vi "4Pi Focus Lock_ids.vi"() -> ()   [LabVIEW 2016]
uses:
  4Pi Focus Lock Controls/4Pi Focus Lock - Notifier Type.ctl
  4Pi Focus Lock Controls/4Pi Focus Lock - Actions.ctl
  <vilib>/vision/Image Controls.llb/IMAQ Image.ctl
  Hardware Configuration/Hardware Configuration Controls/Device Type.ctl
  Hardware Configuration/Hardware Configuration Controls/Device Function.ctl
  Device Library/Cameras/Camera Controls/Generic Camera ROI.ctl
  Device Library/Cameras/Camera Controls/Generic Camera Actions.ctl
  Device Library/Stages/Stages Controls/Stage Actions.ctl
  <vilib>/addons/control/pid/pid.llb/PID (DBL).vi
  <vilib>/addons/control/pid/NI_PID_pid.lvlib
  <vilib>/vision/NI_Vision_Development_Module.lvlib
panel:
  out "CC Max":cluster{" cc max":dbl}(graph)
  in  "Pixe Size (µm)":dbl=1.0
  out "X Y Fit Value (µm)":cluster{dbl, dbl, dbl}(graph)
  out "cc max":dbl=1.0 format="%.3g"
  out "Target X Position cc (px)":dbl=1.0 format="%.3g"
  out "Target Y Position cc (px)":dbl=1.0 format="%.3g"
  out "Measured Y Position cc (px)":dbl=1.0 format="%.3g"
  out "Measured X Position cc (px)":dbl=1.0 format="%.3g"
  in  "Z Correction Active":bool=TRUE
  in  "Frame Accumulation":u32=5
  in  "Z Drift Threshold (µm)":dbl=2.0
  in  "Z Move Limit (µm)":dbl=2.0
  out "Z Move":bool
  in  "Update Scale Factor":dbl=2.0
  out "dz (µm)":dbl format="%.2f"
  out "dt (s)":dbl format="%.3f"
  out "Measured Z (µm)":dbl=1.0 format="%.3g"
  out "Target Z (µm)":dbl=1.0 format="%.3g"
  out "Stage Position (µm)":dbl=1.0 format="%.2g"
  in  "Quit":bool
  in  "Sample Z Step No.":u32=2
  in  "Sample Z Step Size (µm)":dbl=2.0
  in  "D (Derivative)":dbl
  in  "I (Integral)":dbl
  in  "P (Proportional)":dbl=2.0
  in  "Set Camera ROI":bool
  out "Z Target and Fit Value (µm)":T1(graph)
  in  "Start Lock":bool
  # "PID Control Values"
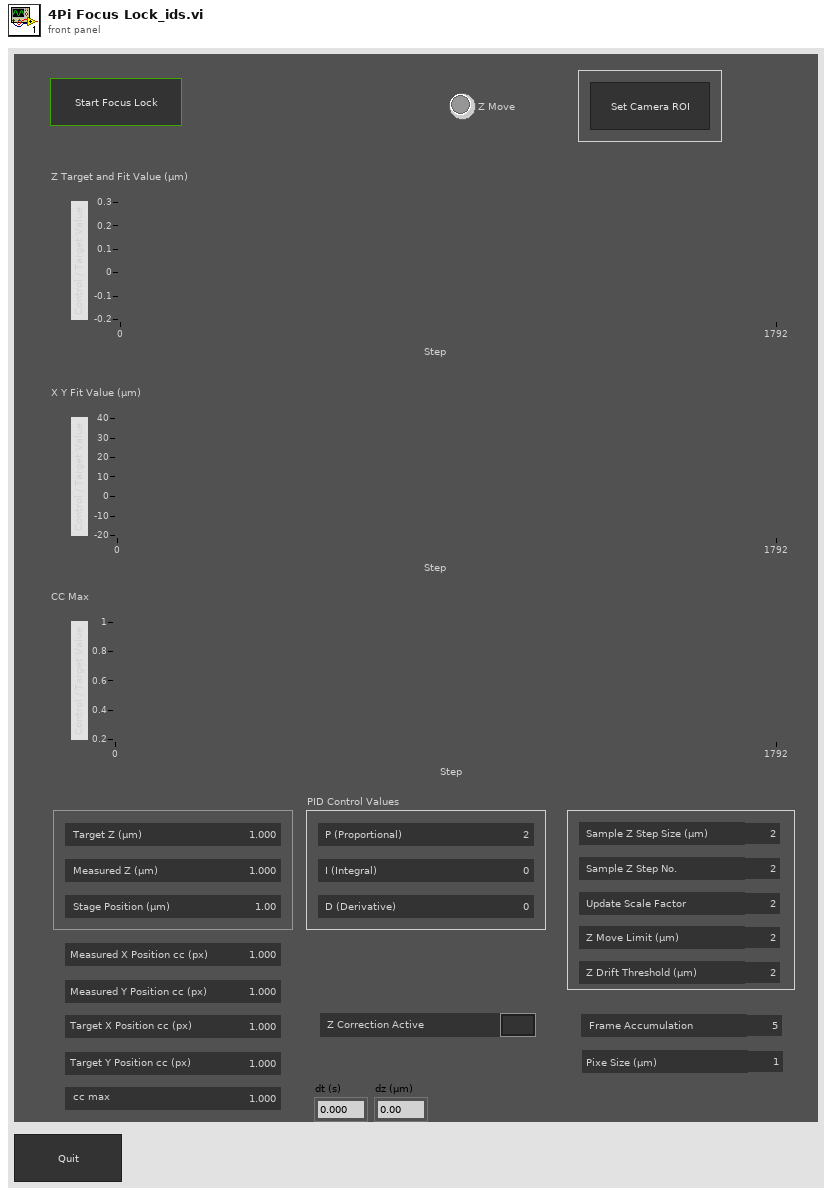
[diagram p1: front panel]
types:
  T1 = cluster{"Target 01":dbl, dbl, dbl, "Current 01":dbl, "Stage Position":dbl}
  T2 = typedef "4Pi Focus Lock - Actions.ctl" = enum16{"Idle", "Start Lock", "Restart Lock", "Get Target Position", "Get Ref Stack", "Cal Ref FFT", "Move To Init Z", "Start Primary Camera", "Get Current Position", "Get Current XY Position", "Get Current Position 1", "Get Actual Position", "Check Drift", "Move Z", "Update Plots", "Delay", "Abort", "Exit Loop", "Quit"}
  T3 = typedef "4Pi Focus Lock - Notifier Type.ctl" = cluster{"Actions":T2, "Z Drift Threshold":dbl, "Z Stage Move Limit (µm)":dbl, "Abort If Error":bool, "Z Correction Active":bool, "PID Values":dbl[], "Running?":bool, "Update Delay (ms)":i32, "Z Step Size (µm)":dbl, "Z Step No.":u32, "No. of Frames":u32, "Ref Stack (SGL)":T4[], "Cur Image (SGL)":T4, "CC Image (SGL) ":T4, "Sample Z (µm)":dbl[], "Initial Z Position (µm)":dbl, "Ref FFT Stack (CSG)":T4[], "Tmp Image FFT (CSG) ":T4[], "CC Image Max (SGL)":T4}
  T4 = typedef "IMAQ Image.ctl" = refnum<image>
  T5 = typedef "Image Type" = u32
  T6 = typedef "Device Function.ctl" = enum16{"Primary", "Secondary", "Overview", "Wide Field Drift Correction", "642 nm Excitation", "560 nm Excitation", "940 nm Excitation", "546 nm Excitation", "488 nm Excitation", "405 nm Excitation", "Objective Drift Correction", "4Pi Focus Lock", "4Pi Objective Lock", "Objective XY", "Objective Z", "Sample XY", "Sample Coarse Z", "Sample Z", "4Pi Lower", "4Pi Upper", "Em Small", "Em Large", "Ex Small", "Ex Large", "Mojo", "Adj Cavity", "Line Scanning", "Alert"}
  T7 = typedef "Device Type.ctl" = enum16{"AOTF", "Camera", "Deformable Mirror", "Laser", "Flip Mirror", "Shutter", "Stage", "Waveform", "FPGA", "Email"}
  T8 = cluster{"Target 01":dbl, dbl, dbl, "Current 01":dbl, "Stage Position":dbl}[]
  T9 = typedef "Stage Actions.ctl" = enum16{"Get Position", "SERVO OFF", "SERVO ON", "SERVO ON/OFF", "MVR", "MOVE", "HALT", "ONTARGET", "ERROR", "REFERENCE", "INIT", "VELOCITY", "STATUS", "EXIT", "HOME", "ZEROPOS", "NANOPOS", "ANALOG", "QUIT"}
  T10 = typedef "Generic Camera Actions.ctl" = enum16{"Status", "Live Preview", "Capture", "Abort", "Set Exposure Time (s)", "Get Exposure Time (s)", "Record Settings", "Set ROI", "Get ROI", "Defect Correction On/Off", "Cooler On/Off", "Fan On/Off", "Quit"}
  T11 = typedef "Generic Camera ROI.ctl" = cluster{"H_Offset":u16, "V_Offset":u16, "H_Width":u16, "V_Width":u16}
  T12 = typedef "Stage Status.ctl" = enum16{"Error", "Abort", "Busy", "On Target"}
  T13 = typedef "2D Gaussian - Best Fit Parameters.ctl" = cluster{"Amplitude":dbl, "X Position":dbl, "Y Position":dbl, "X Width":dbl, "Y Width":dbl, "Offset":dbl}
  T14 = cluster{"PID Values[0]":dbl, "PID Values[1]":dbl, "PID Values[2]":dbl}
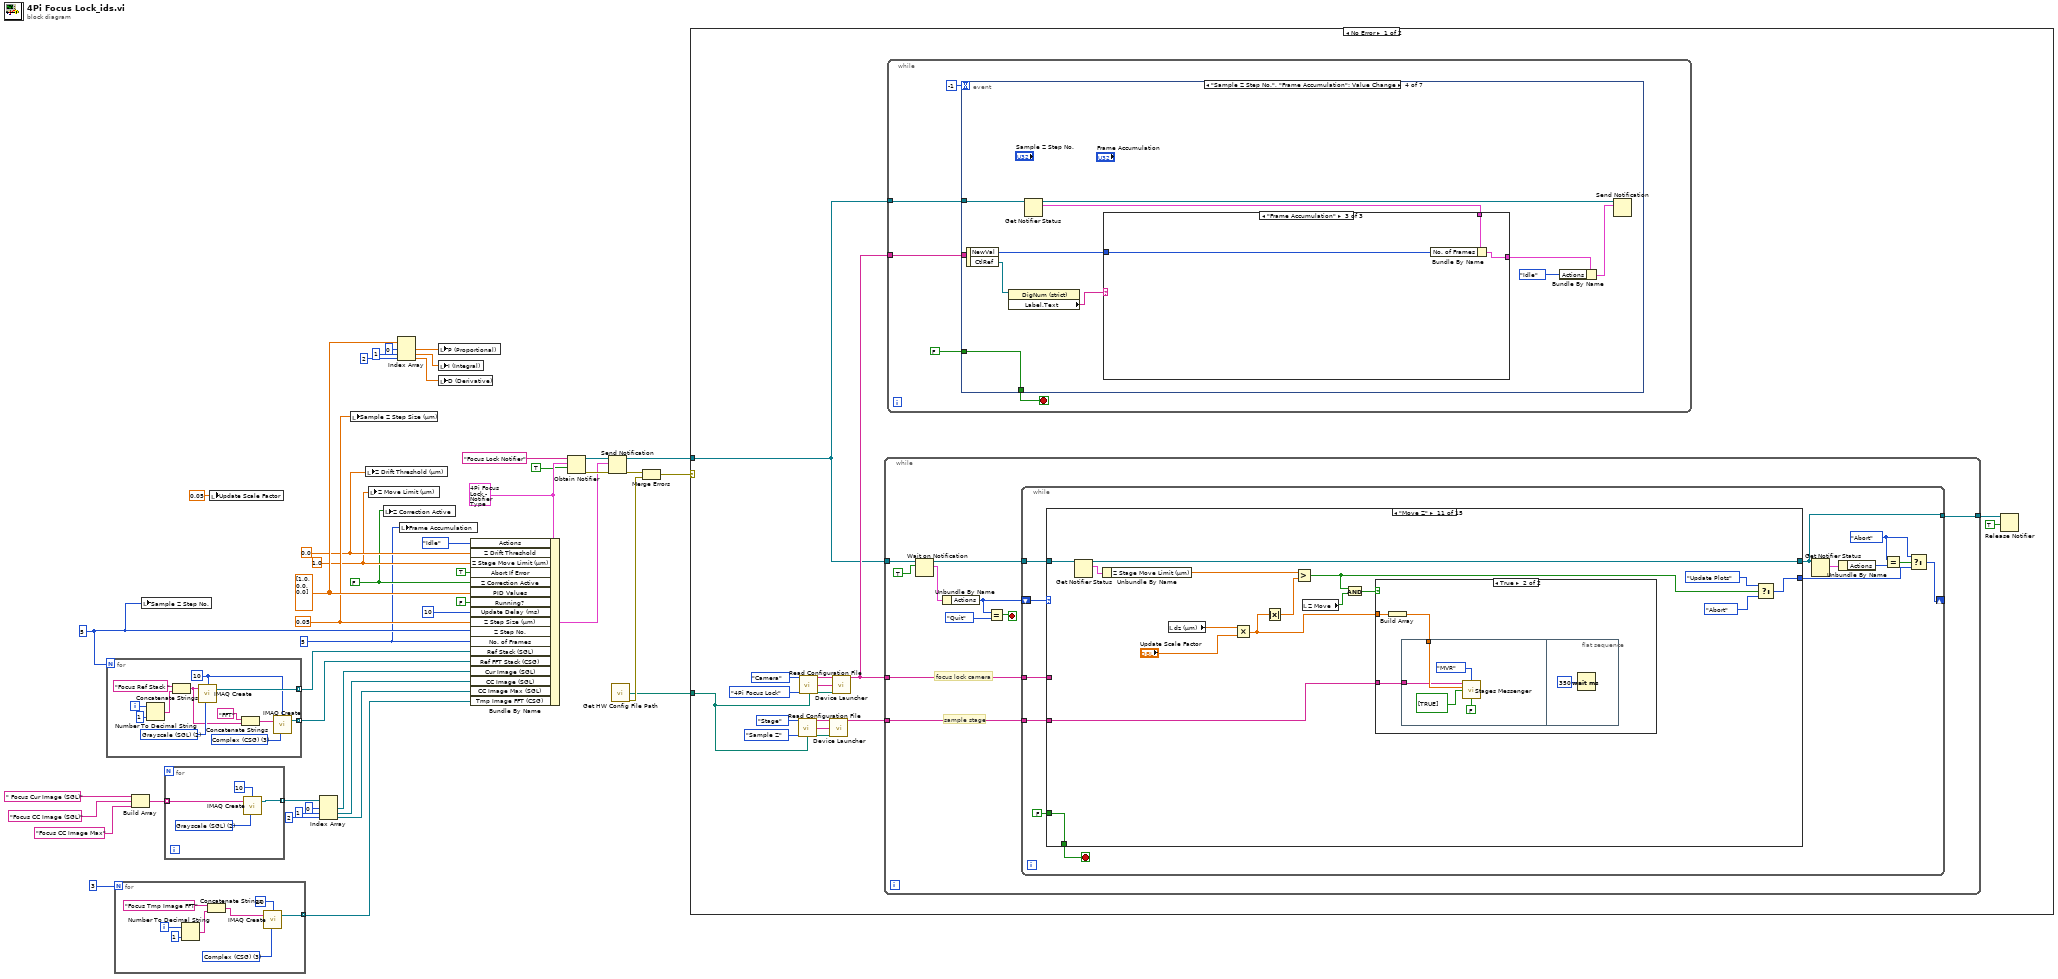
[diagram p0: block diagram]
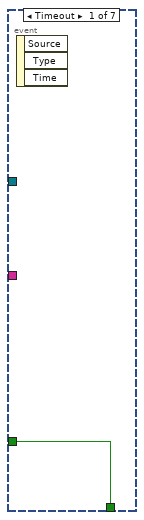
[diagram p2: hidden frame]
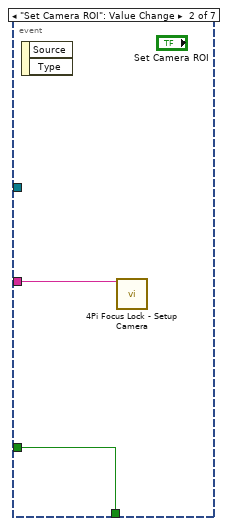
[diagram p3: hidden frame]
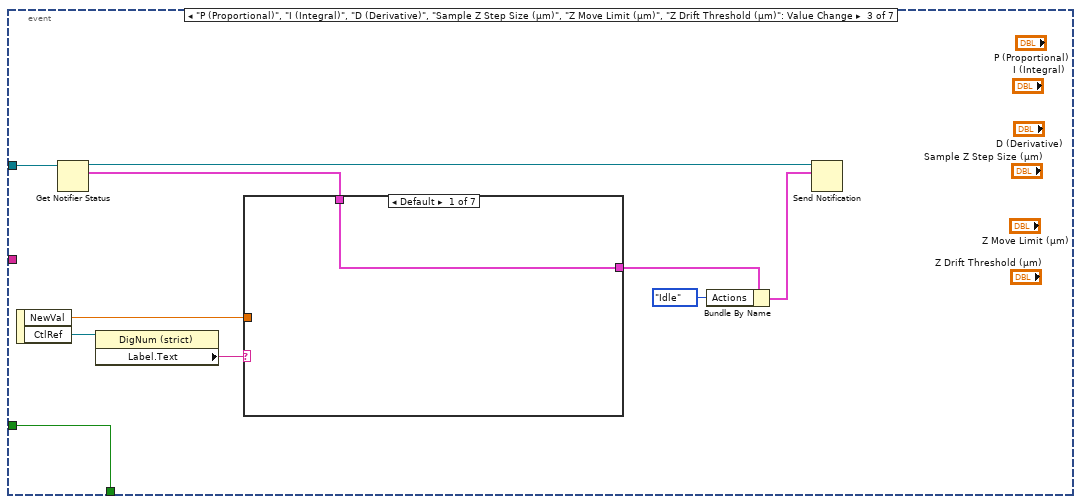
[diagram p4: hidden frame]
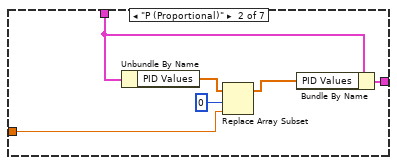
[diagram p5: hidden frame]
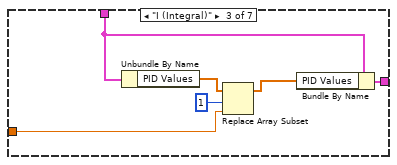
[diagram p6: hidden frame]
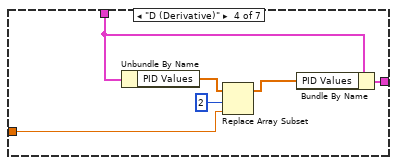
[diagram p7: hidden frame]
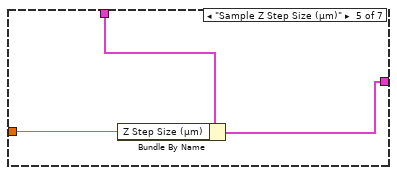
[diagram p8: hidden frame]
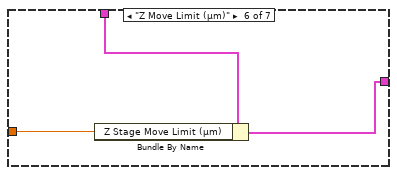
[diagram p9: hidden frame]
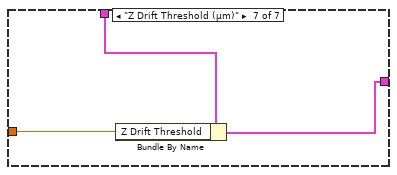
[diagram p10: hidden frame]
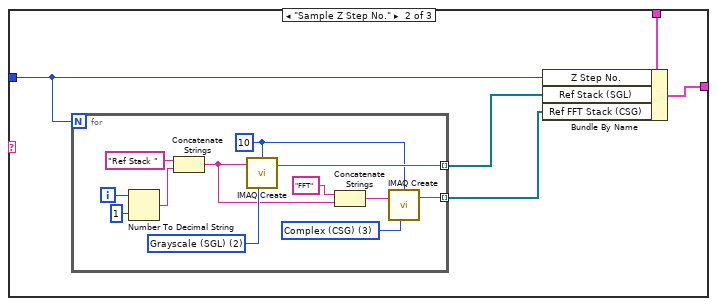
[diagram p12: hidden frame]
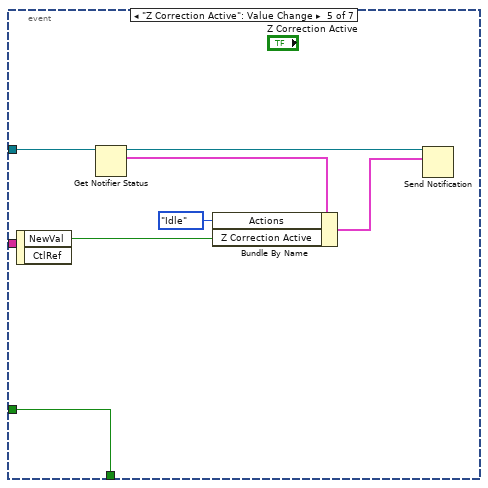
[diagram p13: hidden frame]
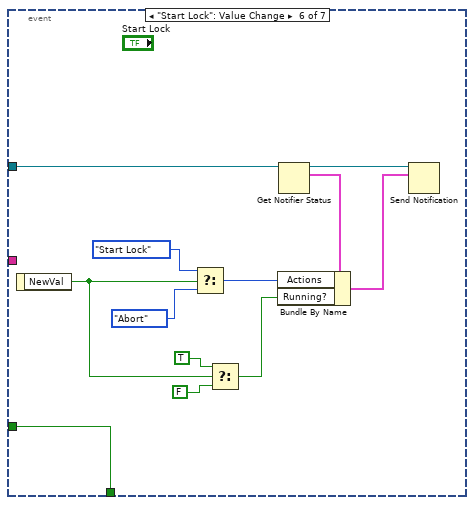
[diagram p14: hidden frame]
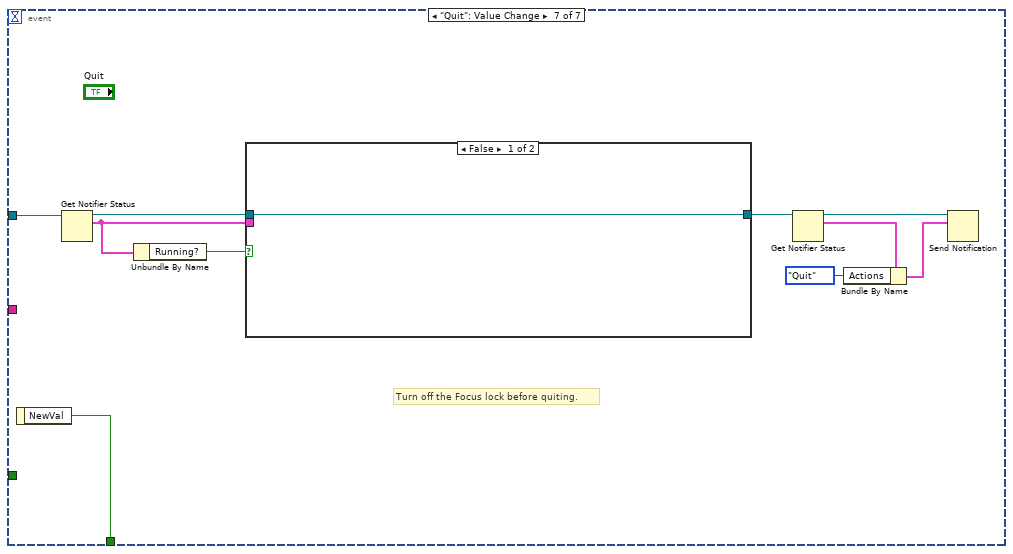
[diagram p15: hidden frame]
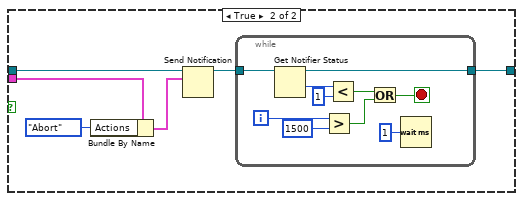
[diagram p16: hidden frame]
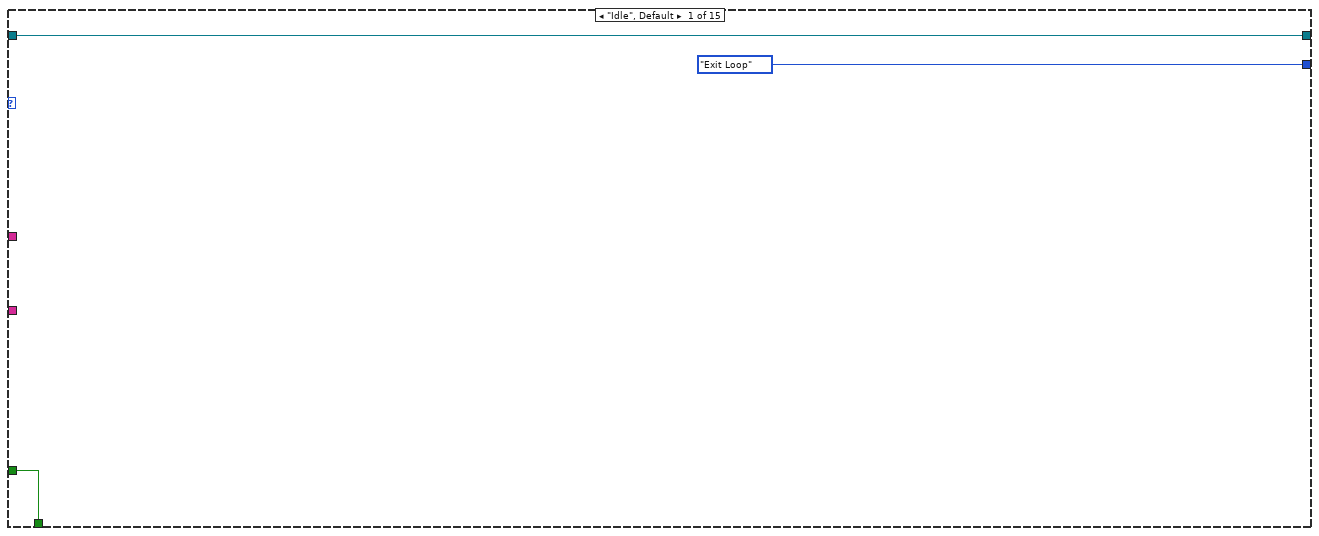
[diagram p17: hidden frame]
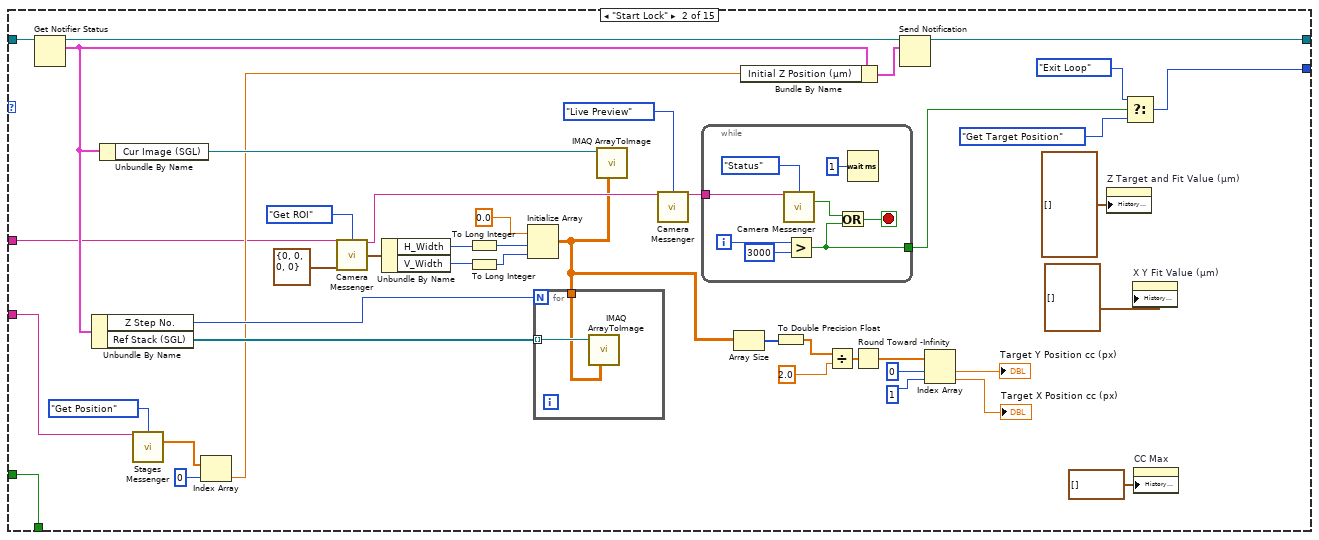
[diagram p18: hidden frame]
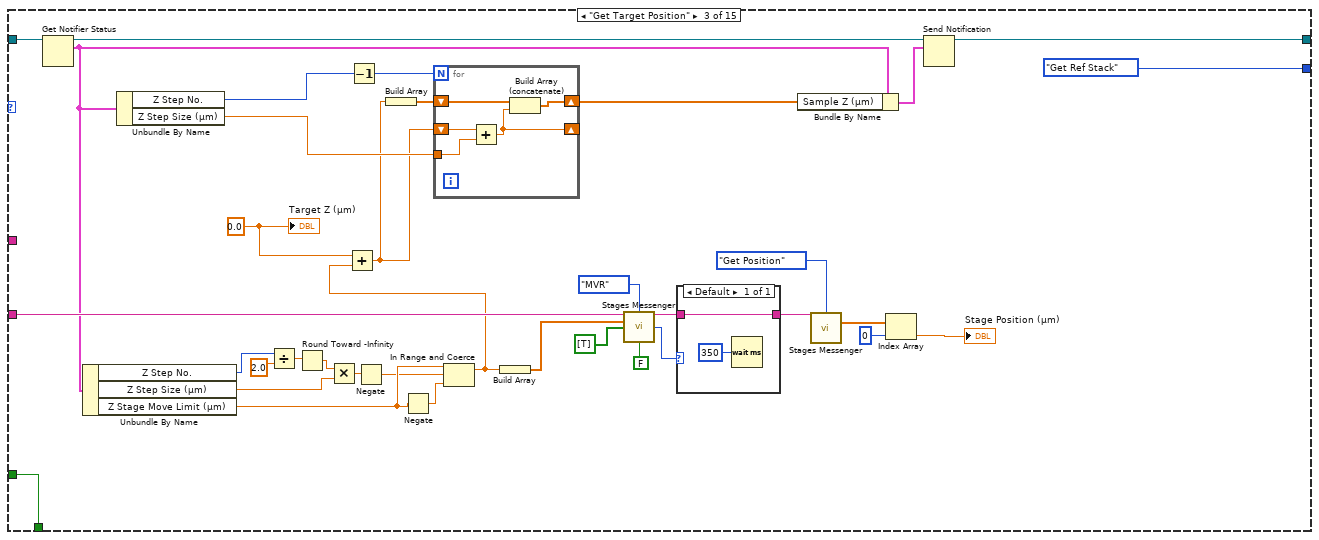
[diagram p19: hidden frame]
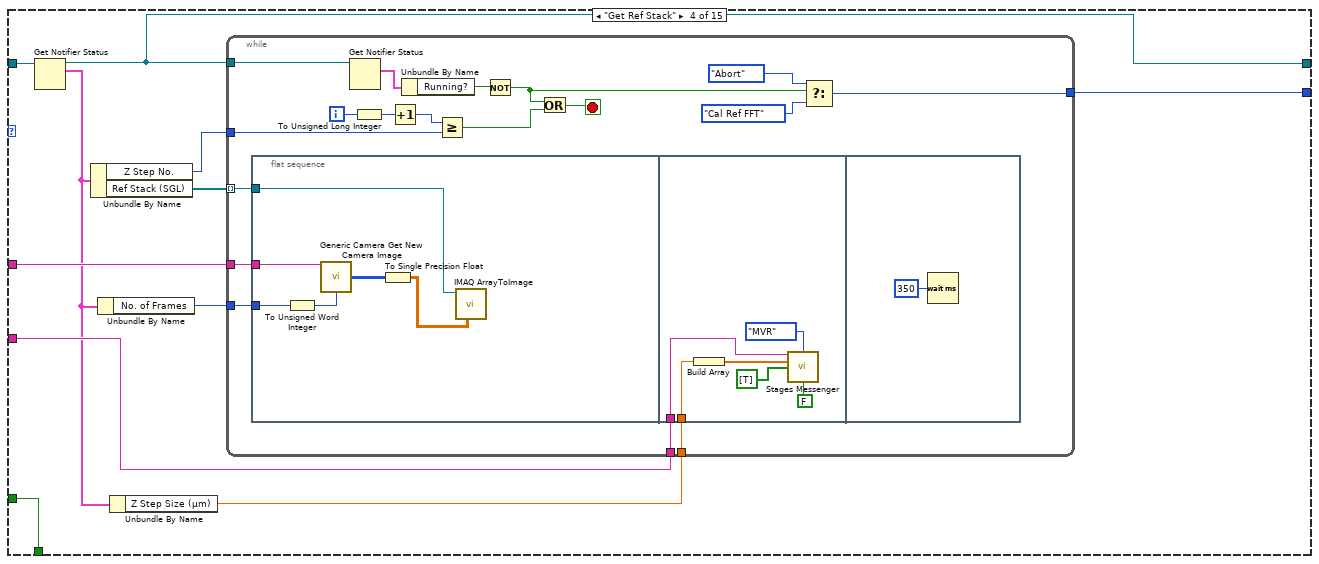
[diagram p20: hidden frame]
diagram:
  w1 = u32 5 ("No. of Frames")
  w24 = u32 5 ("Z Step No.")
  w30 = 0.05 ("Z Step Size (µm)")
  w34 = dbl[] [1.0, 0.0, 0.0] ("PID Values")
  w5 = FALSE ("Z Correction Active")
  w11 = 1.0 ("Z Stage Move Limit (µm)")
  w12 = 0.0 ("Z Drift Threshold")
  w14 = T3 {"Actions"=enum."Idle", "Z Drift Threshold"=0.05, "Z Stage Move Limit (µm)"=1.0, "Abort If Error"=FALSE, "Z Correction Active"=FALSE, "PID Values"=[], "Running?"=FALSE, "Update Delay (ms)"=0, "Z Step Size (µm)"=2.0, "Z Step No."=2, "No. of Frames"=0, "Ref Stack (SGL)"=[], "Cur Image (SGL)"=refnum, "CC Image (SGL) "=refnum, "Sample Z (µm)"=[], "Initial Z Position (µm)"=0.0, "Ref FFT Stack (CSG)"=[], "Tmp Image FFT (CSG) "=[], "CC Image Max (SGL)"=refnum} ("4Pi Focus Lock")
  n1 = for {
    N: w24 -> [_]
    tunnel: [w56] -> w23 mode=indexing
    tunnel: [w45] -> w8 mode=indexing
    i -> [w55]
    w50 = T5 3 items=["Grayscale (U8)", "Grayscale (I16)", "Grayscale (SGL)", "Complex (CSG)", "RGB (U32)", "HSL (U32)", "RGB (U64)", "Grayscale (U16)"] ("Image Type")
    w51 = T5 2 items=["Grayscale (U8)", "Grayscale (I16)", "Grayscale (SGL)", "Complex (CSG)", "RGB (U32)", "HSL (U32)", "RGB (U64)", "Grayscale (U16)"] ("Image Type")
    w47 = 10 ("Border Size")
    n2 = Number To Decimal String(number=w55, width (-)=i16 1) -> (decimal integer string=w53:string)
    n3 = Concatenate Strings("Focus Ref Stack " ("string"), w53) -> (w46:string)
    n4 = call "IMAQ Create"("Border Size"=w47, "Image Name"=w46, "Image Type"=w51) -> ("New Image"=w56:T4)  [unwired: 2 in, 1 out]
    n5 = Concatenate Strings("FFT" ("string"), w46) -> (w49:string)
    n6 = call "IMAQ Create"("Border Size"=w47, "Image Name"=w49, "Image Type"=w50) -> ("New Image"=w45:T4)  [unwired: 2 in, 1 out]
  }
  n7 = for {
    N: 3 -> [_]
    tunnel: [w62] -> w6 mode=indexing
    i -> [w58]
    w63 = T5 3 items=["Grayscale (U8)", "Grayscale (I16)", "Grayscale (SGL)", "Complex (CSG)", "RGB (U32)", "HSL (U32)", "RGB (U64)", "Grayscale (U16)"] ("Image Type")
    n8 = Number To Decimal String(number=w58, width (-)=i16 1) -> (decimal integer string=w61:string)
    n9 = Concatenate Strings("Focus Tmp Image FFT" ("Image Name"), w61) -> (w57:string)
    n10 = call "IMAQ Create"("Border Size"=10, "Image Name"=w57, "Image Type"=w63) -> ("New Image"=w62:T4)  [unwired: 2 in, 1 out]
  }
  n11 = Build Array(" Focus Cur Image (SGL)" ("Image Name"), "Focus CC Image (SGL)" ("Image Name"), "Focus CC Image Max" ("element")) -> (w18:string[])
  n12 = local write "Sample Z Step No."(w24) -> ()
  n13 = for {
    tunnel: w18 -> [w66] mode=indexing
    tunnel: [w65] -> w17 mode=indexing
    w67 = T5 2 items=["Grayscale (U8)", "Grayscale (I16)", "Grayscale (SGL)", "Complex (CSG)", "RGB (U32)", "HSL (U32)", "RGB (U64)", "Grayscale (U16)"] ("Image Type")
    n14 = call "IMAQ Create"("Border Size"=10, "Image Name"=w66, "Image Type"=w67) -> ("New Image"=w65:T4)  [unwired: 2 in, 1 out]
  }
  n15 = local write "Update Scale Factor"(0.05 ("Update Scale Factor")) -> ()
  n16 = Index Array(array=w17, index #1=0 ("index"), index #2=1 ("index"), index #3=2 ("index")) -> (element #1=w16:T4, element #2=w15:T4, element #3=w2:T4)
  n17 = local write "Sample Z Step Size (µm)"(w30) -> ()
  n18 = local write "Z Drift Threshold (µm)"(w12) -> ()
  n19 = local write "Z Move Limit (µm)"(w11) -> ()
  n20 = local write "Z Correction Active"(w5) -> ()
  n21 = Index Array(array=w34, index #1=0 ("index"), index #2=1 ("index"), index #3=2 ("index")) -> (element #1=w33:dbl, element #2=w32:dbl, element #3=w31:dbl)
  n22 = local write "Frame Accumulation"(w1) -> ()
  n23 = local write "P (Proportional)"(w33) -> ()
  n24 = local write "I (Integral)"(w32) -> ()
  n25 = local write "D (Derivative)"(w31) -> ()
  n26 = Bundle By Name(cluster=w14, "Actions"=4Pi_Focus_Lock_-_Actions."Idle", "Z Drift Threshold"=w12, "Z Stage Move Limit (µm)"=w11, "Abort If Error"=TRUE, "Z Correction Active"=w5, "PID Values"=w34, "Running?"=FALSE, "Update Delay (ms)"=10, "Z Step Size (µm)"=w30, "Z Step No."=w24, "No. of Frames"=w1, "Ref Stack (SGL)"=w23, "Ref FFT Stack (CSG)"=w8, "Cur Image (SGL)"=w16, "CC Image (SGL)"=w15, "CC Image Max (SGL)"=w2, "Tmp Image FFT (CSG)"=w6) -> (w9:T3)
  n27 = Obtain Notifier(name (unnamed)="Focus Lock Notifier", notification data type=w14, create if not found? (T)=TRUE) -> (notifier out=w39:refnum<notifier>, error out=w38:errorcluster)  [unwired: 1 in, 1 out]
  n28 = Send Notification(notification=w9, notifier=w39, error in (no error)=w38) -> (notifier out=w25:refnum<notifier>, error out=w29:errorcluster)
  n29 = call "Get HW Config File Path.vi"() -> ("File Path"=w27:path, "Error"=w28:errorcluster)  [unwired: 14 in]
  n30 = Merge Errors(w29, w28) -> (w26:errorcluster)
  n31 = case shown="No Error" w26 {
    tunnel: w27 -> [w69 _]
    tunnel: w25 -> [w72 _]
    frame No Error {
      n32 = call "Read Configuration File.vi"("Device Type"=Device_Type."Stage", "Device Function"=Device_Function."Sample Z", "Config File Path"=w69) -> ("Unique Notifier Name"=w79:string, "Device Ports/IDs/Channels"=w77:string[], "Device Engine Path"=w76:path)  [unwired: 9 in, 1 out]
      n33 = call "Read Configuration File.vi"("Device Type"=Device_Type."Camera", "Device Function"=Device_Function."4Pi Focus Lock", "Config File Path"=w69) -> ("Unique Notifier Name"=w84:string, "Device Ports/IDs/Channels"=w83:string[], "Device Engine Path"=w82:path)  [unwired: 9 in, 1 out]
      n34 = call "Device Launcher.vi"("Notifier Name"=w79, "Device Ports/IDs/Channels"=w77, "Device Engine Path"=w76) -> ("Notifier Name"=w74:string)  [unwired: 11 in, 1 out]
      n35 = call "Device Launcher.vi"("Notifier Name"=w84, "Device Ports/IDs/Channels"=w83, "Device Engine Path"=w82) -> ("Notifier Name"=w73:string)  [unwired: 11 in, 1 out]
      n36 = while {
        tunnel: w72 -> [w217]
        tunnel: w73 -> [w211]
        tunnel: w74 -> [w210]
        tunnel: [w208] -> w70
        stop <- w213 stop-if-true
        # "sample stage"
        # "focus lock camera"
        n37 = Wait on Notification(notifier=w217, ignore previous (F)=TRUE) -> (notifier out=w209:refnum<notifier>, notification=w215:T3)  [unwired: 2 in, 2 out]
        n38 = Unbundle By Name(w215) -> ("Actions"=w212:T2)
        n39 = Equal?(x=w212, y=4Pi_Focus_Lock_-_Actions."Quit") -> (x = y?=w213:bool)
        n40 = while {
          tunnel: w211 -> [w229]
          tunnel: w210 -> [w228]
          tunnel: w209 -> [w227]
          shift-right: [w221] -> _
          shift-left: w212 -> [w230]
          tunnel: [w218] -> w208
          stop <- w220 stop-if-true
          w223 = 4Pi_Focus_Lock_-_Actions."Abort" ("y")
          n41 = case shown="\"Move Z\"" w230 {
            tunnel: w229 -> [_ w253 _ w339 _ _ w425 _ w482 _ _ _ w594 _ _]
            tunnel: w228 -> [_ w260 w317 w332 _ w384 _ _ _ _ w541 w577 _ _ _]
            tunnel: w227 -> [w231 w269 w318 w340 w377 w389 w438 w457 w497 w526 w546 w587 w595 w602 w605]
            tunnel: [4Pi_Focus_Lock_-_Actions."Exit Loop" ("y") w247 4Pi_Focus_Lock_-_Actions."Get Ref Stack" ("y") w333 4Pi_Focus_Lock_-_Actions."Move To Init Z" ("y") 4Pi_Focus_Lock_-_Actions."Get Current Position" ("y") w428 4Pi_Focus_Lock_-_Actions."Check Drift" ("y") 4Pi_Focus_Lock_-_Actions."Check Drift" ("y") w509 w531 4Pi_Focus_Lock_-_Actions."Get Current Position" ("y") 4Pi_Focus_Lock_-_Actions."Exit Loop" ("y") 4Pi_Focus_Lock_-_Actions."Exit Loop" ("y") 4Pi_Focus_Lock_-_Actions."Quit" ("y")] -> w222
            tunnel: [w231 w255 w305 w335 w374 w387 w435 w453 w492 w519 w539 w575 w591 w602 w605] -> w218
            tunnel: [w232 w254 w304 w334 w372 w385 w434 w451 w491 w518 w538 w574 w590 TRUE TRUE] -> w220
            tunnel: FALSE -> [w232 w254 w304 w334 w372 w385 w434 w451 w491 w518 w538 w574 w590 _ _]
            frame "Idle", Default {
            }
            frame "Start Lock" {
              n42 = Get Notifier Status(notifier=w269) -> (notifier out=w256:refnum<notifier>, current notification=w259:T3)  [unwired: 1 in, 3 out]
              n43 = Unbundle By Name(w259) -> ("Z Step No."=w266:u32, "Ref Stack (SGL)"=w265:T4[])
              n44 = Unbundle By Name(w259) -> ("Cur Image (SGL)"=w264:T4)
              n45 = call "Stages Messenger.vi"("Stage Notifier Name"=w260, "Actions"=Stage_Actions."Get Position") -> ("Positions"=w261:dbl[])  [unwired: 9 in, 4 out]
              n46 = Index Array(array=w261, index=0) -> (element=w258:dbl)
              n47 = call "Camera Messenger.vi"("Notifier Name"=w253, "General Camera Actions"=Generic_Camera_Actions."Get ROI", "Camera ROI"=T11 {"H_Offset"=0, "V_Offset"=0, "H_Width"=0, "V_Width"=0} ("General Camera ROI")) -> ("Notifier Name Dup"=w252:string, "Camera ROI"=w274:T11)  [unwired: 7 in, 4 out]
              n48 = Unbundle By Name(w274) -> ("H_Width"=w273:u16, "V_Width"=w271:u16)
              n49 = To Long Integer(number=w273) -> (32bit integer=w272:i32)
              n50 = To Long Integer(number=w271) -> (32bit integer=w270:i32)
              n51 = Initialize Array(sgl 0.0 ("element"), w272, w270) -> (w237:sgl[][])
              n52 = for {
                N: w266 -> [_]
                tunnel: w237 -> [w285]
                tunnel: w265 -> [w286] mode=indexing
                n53 = call "IMAQ ArrayToImage"("Image Pixels (Float)"=w285, "Image"=w286) -> ()  [unwired: 8 in, 2 out]
              }
              n54 = call "IMAQ ArrayToImage"("Image Pixels (Float)"=w237, "Image"=w264) -> ()  [unwired: 8 in, 2 out]
              n55 = call "Camera Messenger.vi"("Notifier Name"=w252, "General Camera Actions"=Generic_Camera_Actions."Live Preview") -> ("Notifier Name Dup"=w251:string)  [unwired: 8 in, 5 out]
              n56 = while {
                tunnel: w251 -> [w283]
                tunnel: [w278] -> w250
                i -> [w282]
                stop <- w279 stop-if-true
                n57 = call "Camera Messenger.vi"("Notifier Name"=w283, "General Camera Actions"=Generic_Camera_Actions."Status") -> ("Running?"=w280:bool)  [unwired: 8 in, 5 out]
                n58 = Greater?(x=w282, y=3000) -> (0:w278:bool)
                n59 = Or(x=w280, y=w278) -> (x .or. y?=w279:bool)
                n60 = Wait (ms)(milliseconds to wait=u32 1) -> ()  [unwired: 1 out]
              }
              n61 = Array Size(array=w237) -> (size(s)=w243:i32[])
              n62 = Bundle By Name(cluster=w259, "Initial Z Position (µm)"=w258) -> (w257:T3)
              n63 = To Double Precision Float(number=w243) -> (double precision float=w246:dbl[])
              n64 = Divide(x=w246, y=2.0 ("index")) -> (x/y=w244:dbl[])
              n65 = Round Toward -Infinity(1:w244) -> (0:w242:dbl[])
              n66 = Send Notification(notification=w257, notifier=w256) -> (notifier out=w255:refnum<notifier>)  [unwired: 1 in, 1 out]
              n67 = Index Array(array=w242, index #1=0 ("index"), index #2=1 ("index")) -> (element #1=→"Target Y Position cc (px)":dbl, element #2=→"Target X Position cc (px)":dbl)
              n68 = property on="Z Target and Fit Value (µm)" class="WFChart (strict)"("History Data"=T8 []) -> ()  [unwired: 2 in, 2 out]
              n69 = Select(t=4Pi_Focus_Lock_-_Actions."Exit Loop" ("y"), s=w250, f=4Pi_Focus_Lock_-_Actions."Get Target Position") -> (s? t:f=w247:T2)
              n70 = property on="X Y Fit Value (µm)" class="WFChart (strict)"("History Data"=cluster{dbl, dbl, dbl}[] []) -> ()  [unwired: 2 in, 2 out]
              n71 = property on="CC Max" class="WFChart (strict)"("History Data"=cluster{" cc max":dbl}[] []) -> ()  [unwired: 2 in, 2 out]
            }
            frame "Get Target Position" {
              w311 = 0.0 ("Target Z (µm)")
              n72 = Get Notifier Status(notifier=w318) -> (notifier out=w309:refnum<notifier>, current notification=w314:T3)  [unwired: 1 in, 3 out]
              n73 = Unbundle By Name(w314) -> ("Z Step No."=w303:u32, "Z Step Size (µm)"=w302:dbl, "Z Stage Move Limit (µm)"=w300:dbl)
              n74 = Unbundle By Name(w314) -> ("Z Step No."=w295:u32, "Z Step Size (µm)"=w312:dbl)
              n75 = Divide(x=w303, y=2.0) -> (x/y=w293:dbl)
              n76 = Round Toward -Infinity(1:w293) -> (0:w292:dbl)
              n77 = Multiply(x=w292, y=w302) -> (x*y=w297:dbl)
              n78 = Decrement(x=w295) -> (x-1=w294:u32)
              n79 = Negate(x=w297) -> (-x=w296:dbl)
              n80 = Negate(x=w300) -> (-x=w301:dbl)
              n81 = In Range and Coerce(upper limit=w300, x=w296, lower limit=w301) -> (coerced(x)=w298:dbl)  [unwired: 1 out]
              n82 = Add(x=w311, y=w298) -> (x+y=w299:dbl)
              n83 = Build Array(w299) -> (w313:dbl[])
              n84 = for {
                N: w294 -> [_]
                tunnel: w312 -> [w327]
                shift-right: [w328] -> w310
                shift-left: w313 -> [w329]
                shift-right: [w325] -> _
                shift-left: w299 -> [w326]
                n85 = Add(x=w326, y=w327) -> (x+y=w325:dbl)
                n86 = Build Array (concatenate)(w329, w325) -> (w328:dbl[])
              }
              n87 = Build Array(w298) -> (w315:dbl[])
              n88 = call "Stages Messenger.vi"("Stage Notifier Name"=w317, "Actions"=Stage_Actions."MVR", "Setpoint"=w315, "Axis"=bool[] [TRUE], "Exit While Busy?"=FALSE) -> ("Stage Notifier Name (Dup)"=w290:string, "Status"=w291:T12)  [unwired: 6 in, 3 out]
              n89 = case shown="Default" w291 {
                tunnel: [w323] -> w289
                tunnel: w290 -> [w323]
                frame Default {
                  n90 = Wait (ms)(milliseconds to wait=u32 350) -> ()  [unwired: 1 out]
                }
              }
              n91 = Bundle By Name(cluster=w314, "Sample Z (µm)"=w310) -> (w308:T3)
              n92 = call "Stages Messenger.vi"("Stage Notifier Name"=w289, "Actions"=Stage_Actions."Get Position") -> ("Positions"=w287:dbl[])  [unwired: 9 in, 4 out]
              n93 = Index Array(array=w287, index=0) -> (element=→"Stage Position (µm)":dbl)
              n94 = Send Notification(notification=w308, notifier=w309) -> (notifier out=w305:refnum<notifier>)  [unwired: 1 in, 1 out]
              "Target Z (µm)" <- w311
            }
            frame "Get Ref Stack" {
              n95 = Get Notifier Status(notifier=w340) -> (notifier out=w335:refnum<notifier>, current notification=w331:T3)  [unwired: 1 in, 3 out]
              n96 = Unbundle By Name(w331) -> ("Z Step No."=w338:u32, "Ref Stack (SGL)"=w337:T4[])
              n97 = Unbundle By Name(w331) -> ("No. of Frames"=w330:u32)
              n98 = Unbundle By Name(w331) -> ("Z Step Size (µm)"=w336:dbl)
              n99 = while {
                tunnel: w339 -> [w358]
                tunnel: w338 -> [w355]
                tunnel: w335 -> [w357]
                tunnel: [w345] -> w333
                tunnel: w337 -> [w344] mode=indexing
                tunnel: w336 -> [w343]
                tunnel: w332 -> [w342]
                tunnel: w330 -> [w341]
                i -> [w354]
                stop <- w350 stop-if-true
                n100 = flat-sequence {
                  tunnel: w358 -> [w362]
                  tunnel: w344 -> [w361]
                  tunnel: w341 -> [w360]
                  tunnel: w343 -> [w366]
                  tunnel: w342 -> [w365]
                  frame #0 {
                    n101 = To Unsigned Word Integer(number=w360) -> (unsigned 16bit integer=w359:u16)
                    n102 = call "Generic Camera Get New Camera Image.vi"("Camera Notifier Name"=w362, "Frames"=w359) -> ("Image - U16"=w364:u16[][])  [unwired: 11 in, 2 out]
                    n103 = To Single Precision Float(number=w364) -> (single precision float=w363:sgl[][])
                    n104 = call "IMAQ ArrayToImage"("Image Pixels (Float)"=w363, "Image"=w361) -> ()  [unwired: 8 in, 2 out]
                  }
                  frame #1 {
                    n105 = Build Array(w366) -> (w370:dbl[])
                    n106 = call "Stages Messenger.vi"("Stage Notifier Name"=w365, "Actions"=Stage_Actions."MVR", "Setpoint"=w370, "Axis"=bool[] [TRUE], "Exit While Busy?"=FALSE) -> ()  [unwired: 6 in, 5 out]
                  }
                  frame #2 {
                    n107 = Wait (ms)(milliseconds to wait=u32 350) -> ()  [unwired: 1 out]
                  }
                }
                n108 = Get Notifier Status(notifier=w357) -> (current notification=w349:T3)  [unwired: 1 in, 4 out]
                n109 = To Unsigned Long Integer(number=w354) -> (unsigned 32bit integer=w353:u32)
                n110 = Increment(x=w353) -> (x+1=w356:u32)
                n111 = Unbundle By Name(w349) -> ("Running?"=w352:bool)
                n112 = Greater Or Equal?(x=w356, y=w355) -> (x >= y?=w351:bool)
                n113 = Not(x=w352) -> (.not. x?=w348:bool)
                n114 = Or(x=w348, y=w351) -> (x .or. y?=w350:bool)
                n115 = Select(t=4Pi_Focus_Lock_-_Actions."Abort", s=w348, f=4Pi_Focus_Lock_-_Actions."Cal Ref FFT" ("y")) -> (s? t:f=w345:T2)
              }
            }
            frame "Cal Ref FFT" {
              n116 = Get Notifier Status(notifier=w377) -> (notifier out=w374:refnum<notifier>, current notification=w378:T3)  [unwired: 1 in, 3 out]
              n117 = Unbundle By Name(w378) -> ("Ref Stack (SGL)"=w375:T4[], "Ref FFT Stack (CSG)"=w376:T4[])
              n118 = for {
                tunnel: w376 -> [w379] mode=indexing
                tunnel: w375 -> [w380] mode=indexing
                n119 = call "4Pi Focus Lock - Norm FFT.vi"("FFT Image Dst"=w379, "Image In"=w380) -> ()  [unwired: 8 in, 2 out]
              }
            }
            frame "Move To Init Z" {
              n120 = Get Notifier Status(notifier=w389) -> (notifier out=w387:refnum<notifier>, current notification=w388:T3)  [unwired: 1 in, 3 out]
              n121 = Unbundle By Name(w388) -> ("Initial Z Position (µm)"=w382:dbl)
              n122 = flat-sequence {
                tunnel: w384 -> [w397]
                tunnel: [w396] -> w383
                tunnel: w382 -> [w392]
                tunnel: [w390] -> w381
                tunnel: w383 -> [w400]
                tunnel: w381 -> [w399]
                frame #0 {
                  n123 = call "Stages Messenger.vi"("Stage Notifier Name"=w397, "Actions"=Stage_Actions."Get Position") -> ("Stage Notifier Name (Dup)"=w396:string, "Positions"=w394:dbl[])  [unwired: 9 in, 3 out]
                  n124 = Index Array(array=w394, index=0) -> (element=w393:dbl)
                  n125 = Subtract(x=w392, y=w393) -> (x-y=w391:dbl)
                  n126 = Build Array(w391) -> (w390:dbl[])
                }
                frame #1 {
                  n127 = call "Stages Messenger.vi"("Stage Notifier Name"=w400, "Actions"=Stage_Actions."MVR", "Setpoint"=w399, "Axis"=bool[] [TRUE], "Exit While Busy?"=FALSE) -> ()  [unwired: 6 in, 5 out]
                }
                frame #2 {
                  n128 = Wait (ms)(milliseconds to wait=u32 350) -> ()  [unwired: 1 out]
                }
              }
            }
            frame "Get Current Position" {
              n129 = Get Notifier Status(notifier=w438) -> (notifier out=w435:refnum<notifier>, current notification=w422:T3)  [unwired: 1 in, 3 out]
              n130 = Unbundle By Name(w422) -> ("CC Image (SGL)"=w410:T4, "CC Image Max (SGL)"=w405:T4)
              n131 = Unbundle By Name(w422) -> ("Ref FFT Stack (CSG)"=w413:T4[])
              n132 = Unbundle By Name(w422) -> ("No. of Frames"=w416:u32, "Cur Image (SGL)"=w424:T4, "Tmp Image FFT (CSG)"=w418:T4[])
              n133 = Unbundle By Name(w422) -> ("Sample Z (µm)"=w437:dbl[])
              n134 = To Unsigned Word Integer(number=w416) -> (unsigned 16bit integer=w415:u16)
              n135 = call "Generic Camera Get New Camera Image.vi"("Camera Notifier Name"=w425, "Frames"=w415) -> ("Image - U16"=w427:u16[][])  [unwired: 11 in, 2 out]
              n136 = Index Array(array=w418, index #1=0 ("index"), index #2=1 ("index"), index #3=2 ("index")) -> (element #1=w417:T4, element #2=w414:T4, element #3=w411:T4)
              n137 = To Single Precision Float(number=w427) -> (single precision float=w426:sgl[][])
              n138 = call "IMAQ ArrayToImage"("Image Pixels (Float)"=w426, "Image"=w424) -> ("Image Out"=w423:T4)  [unwired: 8 in, 1 out]
              n139 = call "4Pi Focus Lock - Norm FFT.vi"("FFT Image Dst"=w417, "Image In"=w423) -> ("FFT Image Out"=w433:T4)  [unwired: 8 in, 1 out]
              n140 = call "IMAQ ComplexConjugate"("Image Src"=w433) -> ("Image Dst Out"=w412:T4)  [unwired: 3 in, 1 out]
              n141 = for {
                tunnel: [w446] -> w408 mode=indexing
                shift-right: [w446] -> _
                shift-left: sgl 0.0 ("Max CC") -> [w447]
                tunnel: w410 -> [w440]
                tunnel: w414 -> [w444]
                tunnel: w413 -> [w443] mode=indexing
                tunnel: w412 -> [w442]
                tunnel: w411 -> [w441]
                tunnel: w405 -> [w439]
                n142 = call "4Pi Focus Lock - Get Cross Correlation.vi"("Ref FFT image"=w443, "Cur FFT Image"=w442, "FFT CC image"=w444, "iFFT image"=w441, "CC image"=w440) -> ("Max CC"=w446:sgl, "CC Image Out"=w445:T4)  [unwired: 8 in, 1 out]
                n143 = Greater?(x=w446, y=w447) -> (0:w448:bool)
                n144 = case shown="True" w448 {
                  tunnel: w439 -> [_ w450]
                  tunnel: w445 -> [_ w449]
                  frame False {
                  }
                  frame True {
                    n145 = call "IMAQ Copy"("Image Dst"=w450, "Image Src"=w449) -> ()  [unwired: 4 in, 2 out]
                  }
                }
              }
              n146 = To Double Precision Float(number=w408) -> (double precision float=w407:dbl[])
              n147 = call "4Pi Focus Lock - Find Peak Position.vi"("Fit Size"=2, "y"=w407, "x"=w437) -> ("Peak value"=→"cc max":dbl, "Coerced Peak Position"=w432:dbl)  [unwired: 6 in, 1 out]
              "Measured Z (µm)" <- w432
              n148 = Not A Number/Path/Refnum?(number/path/refnum=w432) -> (NaN/Path/Refnum?=w431:bool)
              n149 = Select(t=4Pi_Focus_Lock_-_Actions."Get Current Position", s=w431, f=4Pi_Focus_Lock_-_Actions."Get Current XY Position" ("y")) -> (s? t:f=w428:T2)
            }
            frame "Get Current XY Position" {
              w467 = 3 ("edge size")
              n150 = Get Notifier Status(notifier=w457) -> (notifier out=w453:refnum<notifier>, current notification=w456:T3)  [unwired: 1 in, 3 out]
              n151 = Unbundle By Name(w456) -> ("CC Image Max (SGL)"=w477:T4)
              n152 = call "IMAQ ImageToArray"("Image"=w477) -> ("Image Pixels (Float)"=w464:sgl[][])  [unwired: 3 in, 4 out]
              n153 = call "4Pi Focus Lock - FFT shift 2D.vi"("Input image"=w464) -> ("fft shifted image"=w463:sgl[][])  [unwired: 10 in]
              n154 = call "4Pi Focus Lock - Crop Imag at Max.vi"("edge size"=w467, "Input array"=w463) -> ("Y"=w473:i32, "X"=w474:i32, "subarray"=w476:sgl[][])  [unwired: 6 in, 1 out]
              n155 = To Double Precision Float(number=w476) -> (double precision float=w459:dbl[][])
              n156 = Build Array(w474, w473) -> (w472:i32[])
              n157 = call "4Pi Focus Lock - 2D Gaussian - Fit -init.vi"("Image In (DBL)"=w459, "width"=10.0) -> ("Best Fit Params"=w475:T13)  [unwired: 12 in, 1 out]
              n158 = To Double Precision Float(number=w472) -> (double precision float=w469:dbl[])
              n159 = Unbundle By Name(w475) -> ("X Position"=w471:dbl, "Y Position"=w470:dbl)
              n160 = Build Array(w471, w470) -> (w468:dbl[])
              n161 = To Double Precision Float(number=w467) -> (double precision float=w466:dbl)
              n162 = Subtract(x=w468, y=w466) -> (x-y=w465:dbl[])
              n163 = Add(x=w465, y=w469) -> (x+y=w460:dbl[])
              n164 = Index Array(array=w460, index #1=0 ("index"), index #2=1 ("index")) -> (element #1=→"Measured X Position cc (px)":dbl, element #2=→"Measured Y Position cc (px)":dbl)
            }
            frame "Get Current Position 1" {
              n165 = Get Notifier Status(notifier=w497) -> (notifier out=w492:refnum<notifier>, current notification=w496:T3)  [unwired: 1 in, 3 out]
              n166 = Unbundle By Name(w496) -> ("No. of Frames"=w479:u32, "Cur Image (SGL)"=w481:T4, "CC Image (SGL)"=w487:T4)
              n167 = Unbundle By Name(w496) -> ("Sample Z (µm)"=w495:dbl[])
              n168 = Unbundle By Name(w496) -> ("Ref Stack (SGL)"=w490:T4[])
              n169 = To Unsigned Word Integer(number=w479) -> (unsigned 16bit integer=w478:u16)
              n170 = call "Generic Camera Get New Camera Image.vi"("Camera Notifier Name"=w482, "Frames"=w478) -> ("Image - U16"=w484:u16[][])  [unwired: 11 in, 2 out]
              n171 = To Single Precision Float(number=w484) -> (single precision float=w483:sgl[][])
              n172 = call "IMAQ ArrayToImage"("Image Pixels (Float)"=w483, "Image"=w481) -> ("Image Out"=w480:T4)  [unwired: 8 in, 1 out]
              n173 = call "4Pi Focus Lock - Img Norm.vi"("Image In"=w480) -> ("Image Dst Out"=w488:T4)  [unwired: 9 in, 1 out]
              n174 = for {
                tunnel: w490 -> [w508] mode=indexing
                tunnel: w488 -> [w506]
                tunnel: w487 -> [w505]
                tunnel: [w504] -> w486 mode=indexing
                n175 = call "4Pi Focus Lock - Img Norm.vi"("Image In"=w508) -> ("Image Dst Out"=w507:T4)  [unwired: 9 in, 1 out]
                n176 = call "IMAQ Multiply"("Image Src A"=w507, "Image Dst"=w505, "Image Src B"=w506) -> ("Image Dst Out"=w503:T4)  [unwired: 4 in, 1 out]
                n177 = call "IMAQ ImageToArray"("Image"=w503) -> ("Image Pixels (Float)"=w502:sgl[][])  [unwired: 3 in, 4 out]
                n178 = Add Array Elements(numeric array=w502) -> (sum=w500:sgl)
                n179 = Array Size(array=w502) -> (size(s)=w501:i32[])
                n180 = Multiply Array Elements(1:w501) -> (0:w499:i32)
                n181 = To Double Precision Float(number=w499) -> (double precision float=w498:dbl)
                n182 = Divide(x=w500, y=w498) -> (x/y=w504:dbl)
              }
              n183 = To Double Precision Float(number=w486) -> (double precision float=w489:dbl[])
              n184 = call "4Pi Focus Lock - Find Peak Position.vi"("Fit Size"=2, "y"=w489, "x"=w495) -> ("Coerced Peak Position"=w485:dbl)  [unwired: 6 in, 2 out]
              n185 = local write "Measured Z (µm)"(w485) -> ()
            }
            frame "Check Drift" {
              n186 = Get Notifier Status(notifier=w526) -> (notifier out=w519:refnum<notifier>, current notification=w525:T3)  [unwired: 1 in, 3 out]
              n187 = Unbundle By Name(w525) -> ("Z Correction Active"=w512:bool, "Z Drift Threshold"=w520:dbl, "PID Values"=w524:dbl[])
              n188 = local read "Measured Z (µm)"() -> (w515:dbl)
              n189 = local read "Target Z (µm)"() -> (w516:dbl)
              n190 = Array To Cluster(array=w524) -> (cluster=w523:T14)
              n191 = Subtract(x=w516, y=w515) -> (x-y=w517:dbl)
              n192 = call-poly <vilib>:"PID.vi"("PID gains"=w523, "process variable"=w515, "setpoint"=w516) -> ("dt out (s)"=→"dt (s)":dbl, "output"=→"dz (µm)":dbl)  [unwired: 7 in]
              n193 = Absolute Value(x=w517) -> (abs(x)=w514:dbl)
              n194 = Greater?(x=w514, y=w520) -> (0:w513:bool)
              n195 = And(x=w512, y=w513) -> (x .and. y?=w511:bool)
              n196 = case shown="False" w511 {
                tunnel: [4Pi_Focus_Lock_-_Actions."Update Plots" ("y") 4Pi_Focus_Lock_-_Actions."Move Z" ("y")] -> w509
                tunnel: [FALSE TRUE] -> w510
                frame False {
                }
                frame True {
                }
              }
              "Z Move" <- w510
            }
            frame "Move Z" {
              n197 = Get Notifier Status(notifier=w546) -> (notifier out=w539:refnum<notifier>, current notification=w545:T3)  [unwired: 1 in, 3 out]
              n198 = Unbundle By Name(w545) -> ("Z Stage Move Limit (µm)"=w543:dbl)
              n199 = local read "dz (µm)"() -> (w544:dbl)
              n200 = Multiply(x=w544, y="Update Scale Factor") -> (x*y=w537:dbl)
              n201 = Absolute Value(x=w537) -> (abs(x)=w542:dbl)
              n202 = Greater?(x=w543, y=w542) -> (0:w533:bool)
              n203 = local read "Z Move"() -> (w535:bool)
              n204 = And(x=w533, y=w535) -> (x .and. y?=w536:bool)
              n205 = case shown="True" w536 {
                tunnel: w537 -> [_ w548]
                tunnel: w541 -> [_ w547]
                frame False {
                }
                frame True {
                  n206 = Build Array(w548) -> (w549:dbl[])
                  n207 = flat-sequence {
                    tunnel: w549 -> [w553]
                    tunnel: w547 -> [w551]
                    frame #0 {
                      n208 = call "Stages Messenger.vi"("Stage Notifier Name"=w551, "Actions"=Stage_Actions."MVR", "Setpoint"=w553, "Axis"=bool[] [TRUE], "Exit While Busy?"=FALSE) -> ()  [unwired: 6 in, 5 out]
                    }
                    frame #1 {
                      n209 = Wait (ms)(milliseconds to wait=u32 350) -> ()  [unwired: 1 out]
                    }
                  }
                }
              }
              n210 = Select(t=4Pi_Focus_Lock_-_Actions."Update Plots" ("y"), s=w533, f=4Pi_Focus_Lock_-_Actions."Abort") -> (s? t:f=w531:T2)
            }
            frame "Update Plots" {
              n211 = Get Notifier Status(notifier=w587) -> (notifier out=w575:refnum<notifier>, current notification=w585:T3)  [unwired: 1 in, 3 out]
              n212 = Unbundle By Name(w585) -> ("Z Drift Threshold"=w586:dbl)
              n213 = Unbundle By Name(w585) -> ("Initial Z Position (µm)"=w584:dbl)
              n214 = call "Stages Messenger.vi"("Stage Notifier Name"=w577, "Actions"=Stage_Actions."Get Position", "Exit While Busy?"=TRUE) -> ("Positions"=w578:dbl[])  [unwired: 8 in, 4 out]
              n215 = local read "Measured Z (µm)"() -> (w588:dbl)
              n216 = local read "Target Z (µm)"() -> (w589:dbl)
              n217 = Index Array(array=w578, index=0) -> (element=w576:dbl)
              n218 = local write "Stage Position (µm)"(w576) -> ()
              n219 = Subtract(x=w576, y=w584) -> (x-y=w583:dbl)
              n220 = call "4Pi Focus Lock - Values Organize Plot Data.vi"("Target 01"=w589, "Value Limit"=w586, "Current 01"=w588, "Stage Position"=w583) -> ("output cluster"=→"Z Target and Fit Value (µm)":T1)  [unwired: 11 in]
              n221 = local read "Measured X Position cc (px)"() -> (w567:dbl)
              n222 = local read "Measured Y Position cc (px)"() -> (w566:dbl)
              n223 = local read "Target X Position cc (px)"() -> (w565:dbl)
              n224 = local read "Target Y Position cc (px)"() -> (w564:dbl)
              n225 = Build Array(w567, w566) -> (w571:dbl[])
              n226 = Build Array(w565, w564) -> (w572:dbl[])
              n227 = Subtract(x=w571, y=w572) -> (x-y=w563:dbl[])
              n228 = Multiply(x=w563, y="Pixe Size (µm)") -> (x*y=w570:dbl[])
              n229 = local read "cc max"() -> (w557:dbl)
              n230 = Index Array(array=w570, index #1=0 ("index"), index #2=1 ("index")) -> (element #1=w562:dbl, element #2=w561:dbl)
              n231 = Bundle(w562, w561, 0.0) -> (→"X Y Fit Value (µm)":cluster{dbl, dbl, dbl})  [unwired: 1 in]
              n232 = Bundle("cc max"=w557) -> (→"CC Max":cluster{" cc max":dbl})  [unwired: 1 in]
            }
            frame "Abort" {
              n233 = Get Notifier Status(notifier=w595) -> (notifier out=w600:refnum<notifier>, current notification=w599:T3)  [unwired: 1 in, 3 out]
              n234 = call "Camera Messenger.vi"("Notifier Name"=w594, "General Camera Actions"=Generic_Camera_Actions."Abort") -> ()  [unwired: 8 in, 6 out]
              n235 = Bundle By Name(cluster=w599, "Running?"=FALSE, "Actions"=4Pi_Focus_Lock_-_Actions."Exit Loop") -> (w597:T3)
              n236 = Send Notification(notification=w597, notifier=w600) -> (notifier out=w591:refnum<notifier>)  [unwired: 1 in, 1 out]
            }
            frame "Exit Loop" {
            }
            frame "Quit" {
              n237 = Get Notifier Status(notifier=w605) -> (current notification=w611:T3)  [unwired: 1 in, 4 out]
              n238 = Unbundle By Name(w611) -> ("Ref Stack (SGL)"=w610:T4[], "Cur Image (SGL)"=w609:T4, "Tmp Image FFT (CSG)"=w608:T4[], "CC Image (SGL)"=w607:T4, "Ref FFT Stack (CSG)"=w604:T4[])
              n239 = Build Array (concatenate)(w610, w609, w608, w607, w604) -> (w606:T4[])
              n240 = for {
                tunnel: w606 -> [w614] mode=indexing
                n241 = call "IMAQ Dispose"("Image"=w614) -> ()  [unwired: 5 in, 1 out]
              }
            }
          }
          n242 = Get Notifier Status(notifier=w218) -> (current notification=w226:T3)  [unwired: 1 in, 4 out]
          n243 = Unbundle By Name(w226) -> ("Actions"=w225:T2)
          n244 = Equal?(x=w223, y=w225) -> (x = y?=w224:bool)
          n245 = Select(t=w223, s=w224, f=w222) -> (s? t:f=w221:T2)
        }
      }
      n246 = while {
        tunnel: w73 -> [w89]
        tunnel: w72 -> [w88]
        stop <- w87 stop-if-true
        n247 = event shown="[3] \"Sample Z Step No.\", \"Frame Accumulation\": Value Change" {
          selector: _ -> [_ _ _ _ _ _ _]
          dyn-events: _ -> [_ _ _ _ _ _ _]
          timeout: -1 -> [_ _ _ _ _ _ _]
          tunnel: w89 -> [_ w92 _ _ _ _ _]
          tunnel: w88 -> [_ _ w102 w140 w168 w179 w183]
          tunnel: [w90 w91 w93 w137 w162 w173 w181] -> w87
          tunnel: FALSE ("NewVal") -> [w90 w91 w93 w137 w162 w173 _]
          event Timeout {
            n248 = event-data() -> ()  [unwired: 1 in, 3 out]
          }
          event "Set Camera ROI": Value Change {
            n249 = event-data() -> ()  [unwired: 1 in, 2 out]
            n250 = call "4Pi Focus Lock - Setup Camera.vi"("Camera Notifier Name"=w92) -> ()  [unwired: 14 in, 1 out]
          }
          event "P (Proportional)", "I (Integral)", "D (Derivative)", "Sample Z Step Size (µm)", "Z Move Limit (µm)", "Z Drift Threshold (µm)": Value Change {
            n251 = event-data() -> ("NewVal"=w97:dbl, "CtlRef"=w99:refnum<vi>)  [unwired: 1 in]
            n252 = Get Notifier Status(notifier=w102) -> (notifier out=w101:refnum<notifier>, current notification=w100:T3)  [unwired: 1 in, 3 out]
            n253 = property class="DigNum (strict)"(reference=w99) -> ("Label.Text"=w98:string)  [unwired: 1 in, 2 out]
            n254 = case shown="Default" w98 {
              tunnel: w100 -> [w103 w106 w112 w118 w124 w127 w130]
              tunnel: w97 -> [_ w107 w113 w119 w123 w126 w129]
              tunnel: [w103 w104 w110 w116 w122 w125 w128] -> w96
              frame Default {
              }
              frame "P (Proportional)" {
                n255 = Unbundle By Name(w106) -> ("PID Values"=w108:dbl[])
                n256 = Replace Array Subset(array=w108, new element=w107, index=0) -> (w105:dbl[])
                n257 = Bundle By Name(cluster=w106, "PID Values"=w105) -> (w104:T3)
              }
              frame "I (Integral)" {
                n258 = Unbundle By Name(w112) -> ("PID Values"=w114:dbl[])
                n259 = Replace Array Subset(array=w114, new element=w113, index=1) -> (w111:dbl[])
                n260 = Bundle By Name(cluster=w112, "PID Values"=w111) -> (w110:T3)
              }
              frame "D (Derivative)" {
                n261 = Unbundle By Name(w118) -> ("PID Values"=w120:dbl[])
                n262 = Replace Array Subset(array=w120, new element=w119, index=2) -> (w117:dbl[])
                n263 = Bundle By Name(cluster=w118, "PID Values"=w117) -> (w116:T3)
              }
              frame "Sample Z Step Size (µm)" {
                n264 = Bundle By Name(cluster=w124, "Z Step Size (µm)"=w123) -> (w122:T3)
              }
              frame "Z Move Limit (µm)" {
                n265 = Bundle By Name(cluster=w127, "Z Stage Move Limit (µm)"=w126) -> (w125:T3)
              }
              frame "Z Drift Threshold (µm)" {
                n266 = Bundle By Name(cluster=w130, "Z Drift Threshold"=w129) -> (w128:T3)
              }
            }
            n267 = Bundle By Name(cluster=w96, "Actions"=4Pi_Focus_Lock_-_Actions."Idle") -> (w94:T3)
            n268 = Send Notification(notification=w94, notifier=w101) -> ()  [unwired: 1 in, 2 out]
          }
          event "Sample Z Step No.", "Frame Accumulation": Value Change {
            n269 = event-data() -> ("NewVal"=w136:u32, "CtlRef"=w132:refnum<vi>)  [unwired: 1 in]
            n270 = property class="DigNum (strict)"(reference=w132) -> ("Label.Text"=w131:string)  [unwired: 1 in, 2 out]
            n271 = Get Notifier Status(notifier=w140) -> (notifier out=w138:refnum<notifier>, current notification=w139:T3)  [unwired: 1 in, 3 out]
            n272 = case shown="\"Frame Accumulation\"" w131 {
              tunnel: w139 -> [w141 w146 w161]
              tunnel: [w141 w145 w159] -> w135
              tunnel: w136 -> [_ w144 w160]
              frame Default {
              }
              frame "Sample Z Step No." {
                n273 = for {
                  N: w144 -> [_]
                  tunnel: [w158] -> w143 mode=indexing
                  tunnel: [w147] -> w142 mode=indexing
                  i -> [w157]
                  w148 = T5 3 items=["Grayscale (U8)", "Grayscale (I16)", "Grayscale (SGL)", "Complex (CSG)", "RGB (U32)", "HSL (U32)", "RGB (U64)", "Grayscale (U16)"] ("Image Type")
                  w153 = T5 2 items=["Grayscale (U8)", "Grayscale (I16)", "Grayscale (SGL)", "Complex (CSG)", "RGB (U32)", "HSL (U32)", "RGB (U64)", "Grayscale (U16)"] ("Image Type")
                  w149 = 10 ("Border Size")
                  n274 = Number To Decimal String(number=w157, width (-)=i16 1) -> (decimal integer string=w155:string)
                  n275 = Concatenate Strings("Ref Stack " ("string"), w155) -> (w151:string)
                  n276 = call "IMAQ Create"("Border Size"=w149, "Image Name"=w151, "Image Type"=w153) -> ("New Image"=w158:T4)  [unwired: 2 in, 1 out]
                  n277 = Concatenate Strings("FFT" ("string"), w151) -> (w150:string)
                  n278 = call "IMAQ Create"("Border Size"=w149, "Image Name"=w150, "Image Type"=w148) -> ("New Image"=w147:T4)  [unwired: 2 in, 1 out]
                }
                n279 = Bundle By Name(cluster=w146, "Z Step No."=w144, "Ref Stack (SGL)"=w143, "Ref FFT Stack (CSG)"=w142) -> (w145:T3)
              }
              frame "Frame Accumulation" {
                n280 = Bundle By Name(cluster=w161, "No. of Frames"=w160) -> (w159:T3)
              }
            }
            n281 = Bundle By Name(cluster=w135, "Actions"=4Pi_Focus_Lock_-_Actions."Idle") -> (w133:T3)
            n282 = Send Notification(notification=w133, notifier=w138) -> ()  [unwired: 1 in, 2 out]
          }
          event "Z Correction Active": Value Change {
            n283 = event-data() -> ("NewVal"=w166:bool)  [unwired: 1 in, 1 out]
            n284 = Get Notifier Status(notifier=w168) -> (notifier out=w164:refnum<notifier>, current notification=w167:T3)  [unwired: 1 in, 3 out]
            n285 = Bundle By Name(cluster=w167, "Actions"=4Pi_Focus_Lock_-_Actions."Idle", "Z Correction Active"=w166) -> (w163:T3)
            n286 = Send Notification(notification=w163, notifier=w164) -> ()  [unwired: 1 in, 2 out]
          }
          event "Start Lock": Value Change {
            n287 = event-data() -> ("NewVal"=w171:bool)  [unwired: 1 in]
            n288 = Select(t=4Pi_Focus_Lock_-_Actions."Start Lock", s=w171, f=4Pi_Focus_Lock_-_Actions."Abort" ("t")) -> (s? t:f=w176:T2)
            n289 = Select(t=TRUE ("Running?"), s=w171, f=FALSE) -> (s? t:f=w169:bool)
            n290 = Get Notifier Status(notifier=w179) -> (notifier out=w180:refnum<notifier>, current notification=w178:T3)  [unwired: 1 in, 3 out]
            n291 = Bundle By Name(cluster=w178, "Actions"=w176, "Running?"=w169) -> (w177:T3)
            n292 = Send Notification(notification=w177, notifier=w180) -> ()  [unwired: 1 in, 2 out]
          }
          event "Quit": Value Change {
            # "Turn off the Focus lock before quiting."
            n293 = event-data() -> ("NewVal"=w181:bool)  [unwired: 1 in]
            n294 = Get Notifier Status(notifier=w183) -> (notifier out=w186:refnum<notifier>, current notification=w184:T3)  [unwired: 1 in, 3 out]
            n295 = Unbundle By Name(w184) -> ("Running?"=w187:bool)
            n296 = case shown="False" w187 {
              tunnel: w186 -> [w191 w196]
              tunnel: [w191 w193] -> w185
              tunnel: w184 -> [_ w197]
              frame False {
              }
              frame True {
                n297 = Bundle By Name(cluster=w197, "Actions"=4Pi_Focus_Lock_-_Actions."Abort") -> (w195:T3)
                n298 = Send Notification(notification=w195, notifier=w196) -> (notifier out=w194:refnum<notifier>)  [unwired: 1 in, 1 out]
                n299 = while {
                  tunnel: w194 -> [w207]
                  tunnel: [w202] -> w193
                  i -> [w201]
                  stop <- w203 stop-if-true
                  n300 = Get Notifier Status(notifier=w207) -> (notifier out=w202:refnum<notifier>, # waiting=w206:i32)  [unwired: 1 in, 3 out]
                  n301 = Greater?(x=w201, y=1500) -> (0:w199:bool)
                  n302 = Less?(x=w206, y=1) -> (x < y?=w204:bool)
                  n303 = Or(x=w204, y=w199) -> (x .or. y?=w203:bool)
                  n304 = Wait (ms)(milliseconds to wait=u32 1) -> ()  [unwired: 1 out]
                }
              }
            }
            n305 = Get Notifier Status(notifier=w185) -> (notifier out=w189:refnum<notifier>, current notification=w190:T3)  [unwired: 1 in, 3 out]
            n306 = Bundle By Name(cluster=w190, "Actions"=4Pi_Focus_Lock_-_Actions."Quit") -> (w188:T3)
            n307 = Send Notification(notification=w188, notifier=w189) -> ()  [unwired: 1 in, 2 out]
          }
        }
      }
      n308 = Release Notifier(notifier=w70, force destroy? (F)=TRUE) -> ()  [unwired: 1 in, 3 out]
    }
    frame Error {
    }
  }
